vi "InitUI.vi"(8 "error in (no error)":errorcluster, 11 "View in":refnum<class "View.lvclass">) -> (0 "error out":errorcluster, 3 "View out":refnum<class "View.lvclass">)   [LabVIEW 2020, in "Container.lvlib" / "View.lvclass"]
uses:
  View.lvclass
  View.lvclass/View.ctl
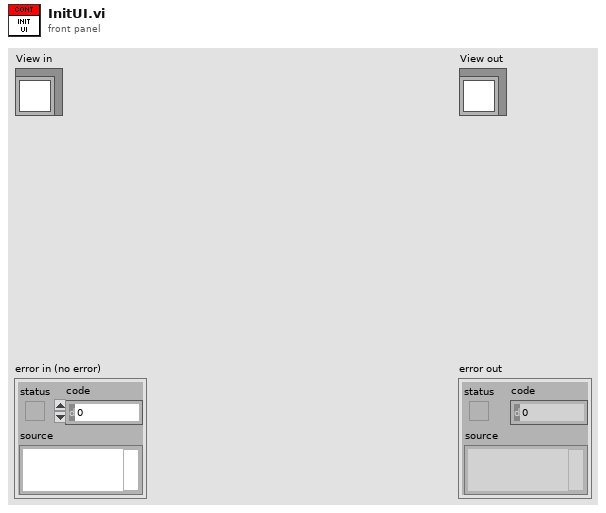
[diagram p1: front panel]
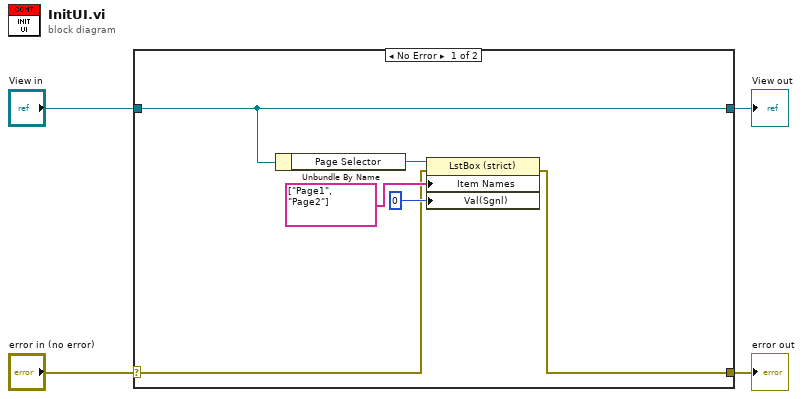
[diagram p0: block diagram]
diagram:
  n1 = case shown="No Error" "error in (no error)" {
    selector: "error in (no error)" -> [w6 w12]
    tunnel: [w5 w12] -> w3
    tunnel: [w8 w11] -> w1
    tunnel: "View in" -> [w8 w11]
    frame No Error {
      n2 = Unbundle By Name(w8) -> ("Page Selector"=w7:refnum<vi>)
      n3 = property class="LstBox (strict)"(reference=w7, error in=w6, "Item Names"=string[] ["Page1", "Page2"], "Val(Sgnl)"=0 ("Value (Signaling)")) -> (error out=w5:errorcluster)  [unwired: 1 out]
    }
    frame Error {
    }
  }
  "error out" <- w3
  "View out" <- w1
